vi "AddSpeedProperty.vi"(8 "error in (no error)":errorcluster, 11 "tdms ref in":refnum<k34>) -> (0 "error out":errorcluster, 3 "tdms ref out":refnum<k34>)   [LabVIEW 2017, in "DataExplorerSupport.lvlib"]
uses:
  <vilib>/addons/InsightCM/Utilities/DataExplorerSupport/DataExplorerSupport.lvlib
  <vilib>/addons/InsightCM/Utilities/Tdms/Tdms.lvlib
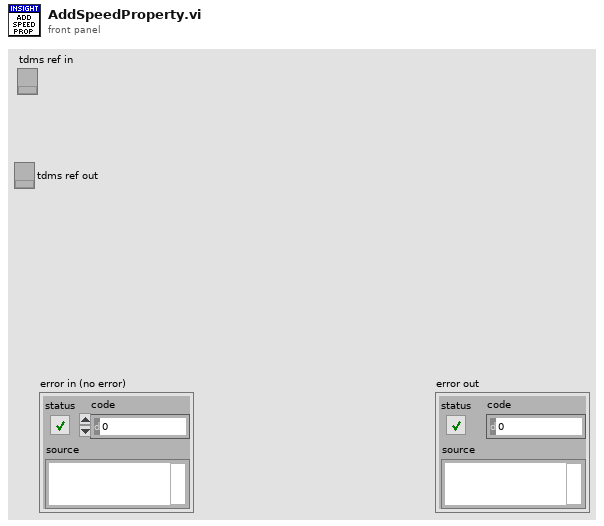
[diagram p1: front panel]
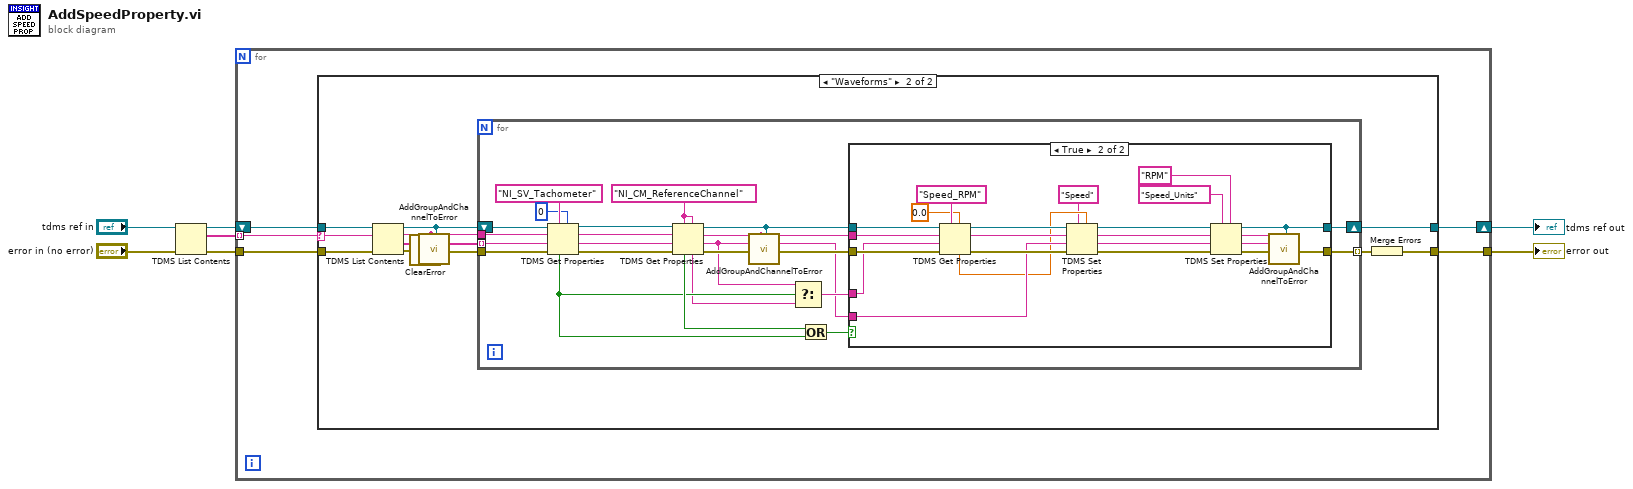
[diagram p0: block diagram]
diagram:
  n1 = TDMS List Contents(4:"error in (no error)", 7:"tdms ref in") -> (0:w2:errorcluster, 2:w1:string[], 3:w4:refnum<k34>)  [unwired: 1 in, 1 out]
  n2 = for {
    tunnel: [w12] -> w7
    tunnel: w2 -> [w9]
    shift-right: [w11] -> w6
    shift-left: w4 -> [w10]
    tunnel: w1 -> [w8] mode=indexing
    n3 = case shown="\"Waveforms\"" w8 {
      selector: w8 -> [_ w15]
      tunnel: [w13 w26] -> w12
      tunnel: [w14 w25] -> w11
      tunnel: w10 -> [w14 w17]
      tunnel: w9 -> [w13 w16]
      frame Default {
      }
      frame "Waveforms" {
        n4 = TDMS List Contents(4:w16, 6:w15, 7:w17) -> (0:w18:errorcluster, 1:w24:string[], 2:w20:string, 3:w19:refnum<k34>)
        n5 = call <vilib>:"ClearError.vi"("error in (no error)"=w18) -> ("error out"=w22:errorcluster)
        n6 = call <vilib>:"AddGroupAndChannelToError.vi"("error in (no error)"=w22, "group name in"=w20, "Refnum in"=w19) -> ("error out"=w21:errorcluster)  [unwired: 16 in]
        n7 = for {
          tunnel: w21 -> [w48]
          tunnel: w20 -> [w44]
          tunnel: w24 -> [w41] mode=indexing
          tunnel: [w33] -> w23 mode=indexing
          shift-right: [w27] -> w25
          shift-left: w19 -> [w45]
          w49 = "NI_CM_ReferenceChannel" ("property name")
          n8 = TDMS Get Properties(5:0 ("number"), 7:"NI_SV_Tachometer" ("property name"), 8:w48, 9:w41, 10:w44, 11:w45) -> (0:w47:errorcluster, 1:w42:string, 2:w43:string, 3:w46:refnum<k34>, 6:w36:bool)  [unwired: 1 out]
          n9 = TDMS Get Properties(5:w49, 7:w49, 8:w47, 9:w42, 10:w43, 11:w46) -> (0:w32:errorcluster, 1:w30:string, 2:w29:string, 3:w28:refnum<k34>, 4:w35:string, 6:w38:bool)
          n10 = call <vilib>:"AddGroupAndChannelToError.vi"("error in (no error)"=w32, "channel name in"=w30, "group name in"=w29, "Refnum in"=w28) -> ("error out"=w31:errorcluster)  [unwired: 15 in]
          n11 = Select(t=w30, s=w36, f=w35) -> (s? t:f=w34:string)
          n12 = Or(x=w38, y=w36) -> (x .or. y?=w37:bool)
          n13 = case shown="True" w37 {
            tunnel: w28 -> [w50 w74]
            tunnel: w31 -> [w51 w73]
            tunnel: w29 -> [_ w72]
            tunnel: w30 -> [_ w68]
            tunnel: [w51 w55] -> w33
            tunnel: w34 -> [_ w57]
            tunnel: [w50 w52] -> w27
            frame False {
            }
            frame True {
              n14 = TDMS Get Properties(5:sgl 0.0, 7:"Speed_RPM" ("property name"), 8:w73, 9:w57, 10:w72, 11:w74) -> (0:w70:errorcluster, 2:w69:string, 3:w71:refnum<k34>, 4:w65:sgl)  [unwired: 2 out]
              n15 = TDMS Set Properties(5:w65, 7:"Speed" ("property names"), 8:w70, 9:w68, 10:w69, 11:w71) -> (0:w62:errorcluster, 1:w61:string, 2:w60:string, 3:w63:refnum<k34>)
              n16 = TDMS Set Properties(5:"RPM" ("property names"), 7:"Speed_Units" ("property names"), 8:w62, 9:w61, 10:w60, 11:w63) -> (0:w56:errorcluster, 1:w54:string, 2:w53:string, 3:w52:refnum<k34>)
              n17 = call <vilib>:"AddGroupAndChannelToError.vi"("error in (no error)"=w56, "channel name in"=w54, "group name in"=w53, "Refnum in"=w52) -> ("error out"=w55:errorcluster)  [unwired: 15 in]
            }
          }
        }
        n18 = Merge Errors(w23) -> (w26:errorcluster)
      }
    }
  }
  "error out" <- w7
  "tdms ref out" <- w6
